vi "test Verify with Multi Scrubber.vi"(8 "error in":errorcluster, 11 "Testing Approval Tests in":refnum<class "VITester Extension Tests.lvclass">) -> (0 "error out":errorcluster, 3 "Testing Approval Tests out":refnum<class "VITester Extension Tests.lvclass">)   [LabVIEW 2020, in "VITester Extension Tests.lvclass"]
uses:
  VITester Extension Tests.lvclass
  Source/Approval Tests/Options.ctl
  Source/Approval Tests/Reporter/Reporter.lvclass
  Source/Approval Tests/Namer/Namer.lvclass
  Source/Approval Tests/Scrubber/Scrubber.lvclass
  Source/Approval Tests/Regex Scrubber/Regex Scrubber.lvclass
  C:/Users/SAS/Desktop/ApprovalTests.LabVIEW/Source/Approval Tests/Scrubber/Scrubber.lvclass
  Source/Approval Tests/Multi Scrubber/Multi Scrubber.lvclass
  Source/Approval Tests/Regex Scrubber/Regex Scrubber.lvclass/Regex Scrubber.ctl
  Source/Approval Tests/Multi Scrubber/Multi Scrubber.lvclass/Multi Scrubber.ctl
  c85dbac9-9df1-4385-95da-0d0c429ccc49.vi
  Source/Approval Tests/Regex Scrubber/Write Regex.vi
  Source/Approval Tests/Regex Scrubber/Write Replacement.vi
  Source/Approval Tests/Multi Scrubber/Write Scrubbers.vi
  c85dbac9-9df1-4385-95da-0d0c429ccc49.vi/ef028380-787c-4fa5-86c8-b0b7860ce2dc.vi
  c85dbac9-9df1-4385-95da-0d0c429ccc49.vi/ef028380-787c-4fa5-86c8-b0b7860ce2dc.vi/93c5622b-9fb7-41e0-8c76-3fde37e94e34.vi
  c85dbac9-9df1-4385-95da-0d0c429ccc49.vi/ef028380-787c-4fa5-86c8-b0b7860ce2dc.vi/93c5622b-9fb7-41e0-8c76-3fde37e94e34.vi/daceb942-e4a5-48f9-868a-a7549e7f6e2f.vi
  Source/Approval Tests/Replace with Caller if Empty.vi
  Source/Approval Tests/conv EOL.vi
  <vilib>/Utility/libraryn.llb/Check if File or Folder Exists.vi
  Source/Approval Tests/Approval Tests.lvlib
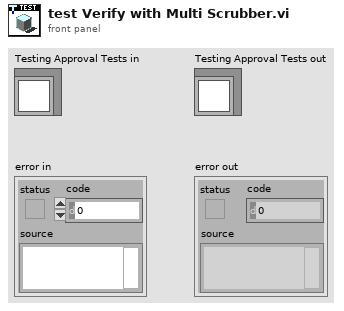
[diagram p1: front panel]
types:
  T1 = typedef "Approval Tests.lvlib/Options.ctl" = cluster{"Reporter":refnum<class "Reporter.lvclass">, "Extension(txt)":string, "Namer":refnum<class "Namer.lvclass">, "Scrubber":refnum<class "Scrubber.lvclass">, "Test Label":string}
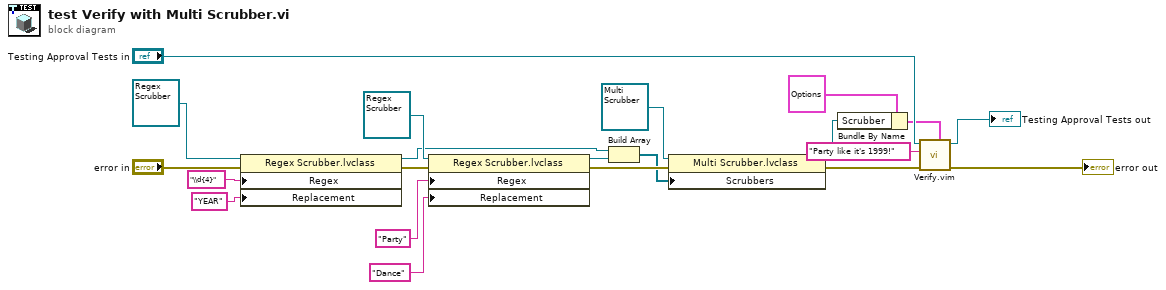
[diagram p0: block diagram]
diagram:
  n1 = property class="Regex Scrubber.lvclass"(reference=refnum<class "Regex Scrubber.lvclass"> refnum ("Approval Tests.lvlib:Regex Scrubber.lvclass"), error in="error in", "Regex"="\\d{4}", "Replacement"="YEAR") -> (reference out=w5:refnum<class "Regex Scrubber.lvclass">, error out=w20:errorcluster)
  n2 = property class="Regex Scrubber.lvclass"(reference=refnum<class "Regex Scrubber.lvclass"> refnum ("Approval Tests.lvlib:Regex Scrubber.lvclass"), error in=w20, "Regex"="Party", "Replacement"="Dance") -> (reference out=w4:refnum<class "Regex Scrubber.lvclass">, error out=w19:errorcluster)
  n3 = Build Array(w5, w4) -> (w3:refnum<class "Regex Scrubber.lvclass">[])
  n4 = property class="Multi Scrubber.lvclass"(reference=refnum<class "Multi Scrubber.lvclass"> refnum ("Approval Tests.lvlib:Multi Scrubber.lvclass"), error in=w19, "Scrubbers"=w3) -> (reference out=w2:refnum<class "Multi Scrubber.lvclass">, error out=w18:errorcluster)
  n5 = Bundle By Name(cluster=T1 {"Reporter"=refnum, "Extension(txt)"="", "Namer"=refnum, "Scrubber"=refnum, "Test Label"=""} ("Options"), "Scrubber"=w2) -> (w13:T1)
  n6 = call "Verify.vim"("Options"=w13, "error in"=w18, "Test Data"="Party like it's 1999!", "TestCase"="Testing Approval Tests in") -> ("error out"=→"error out":errorcluster, "TestCase"=→"Testing Approval Tests out":refnum<class "VITester Extension Tests.lvclass">)  [unwired: 6 in]
